vi "QT7600.vi"() -> ()   [LabVIEW 2015]
panel:
  out "return count 2":u32
  in  "write buffer 2":string
  out "return count":u32
  in  "VISA QT7600":refnum<visa-resource-name>
  in  "write buffer":string
  in  "error in (no error)":errorcluster
  out "VISA out":refnum<visa-resource-name>
  out "read buffer":string
  out "return count 3":u32
  out "error out":errorcluster
  in  "byte count":u32
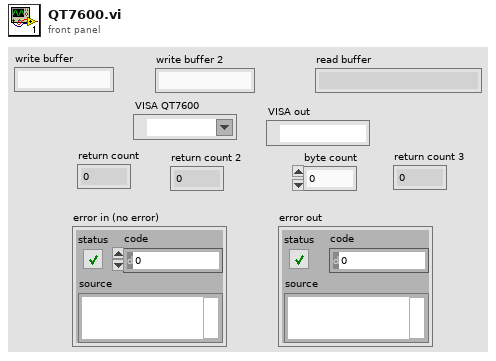
[diagram p1: front panel]
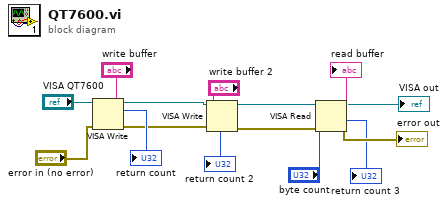
[diagram p0: block diagram]
diagram:
  n1 = VISA Write(VISA resource name="VISA QT7600", write buffer="write buffer", error in (no error)="error in (no error)") -> (VISA resource name out=w2:refnum<visa-resource-name>, return count=→"return count":u32, error out=w4:errorcluster)
  n2 = VISA Write(VISA resource name=w2, write buffer="write buffer 2", error in (no error)=w4) -> (VISA resource name out=w1:refnum<visa-resource-name>, return count=→"return count 2":u32, error out=w3:errorcluster)
  n3 = VISA Read(VISA resource name=w1, byte count="byte count", error in (no error)=w3) -> (VISA resource name out=→"VISA out":refnum<visa-resource-name>, read buffer=→"read buffer":string, return count=→"return count 3":u32, error out=→"error out":errorcluster)
